vi "Patrick-UTiLIA-Lock.vi"(2 "Reset Filter?":bool, 3 "Sampling Info":cluster{"Fs":dbl[unit], "#S":i32}={"Fs"=55872.0, "#S"=8192}, 4 "Cutoff Freq":dbl[unit]=0.9 format="%.2f", 5 "Filter Type":T1(ring)=enum."Chebyshev", 6 "Unit Reference":dbl[](array[numeric]) format="%.2f", 7 "Noisy Signal":dbl[](array[numeric]) format="%.2f") -> (0 "Multiplied Signal":dbl[](array[numeric]) format="%.2f", 1 "Locked Signal":dbl[](array[numeric]) format="%.2f")   [LabVIEW 2013]
uses:
  <vilib>/Analysis/3filter.llb/Butterworth Filter (DBL).vi
  <vilib>/Analysis/3filter.llb/Chebyshev Filter (DBL).vi
  <vilib>/Analysis/3filter.llb/Inverse Chebyshev Filter (DBL).vi
  <vilib>/Analysis/NI_AALBase.lvlib
panel:
  in  "Attenuation(dB)":dbl=120.0 format="%.2f"
  in  "Filter Order":i32=10
  in  "Passband Ripple(dB)":dbl=0.1 format="%.2f"
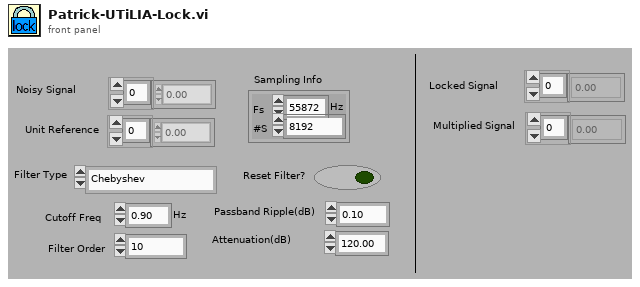
[diagram p1: front panel]
types:
  T1 = enum16{"None", "Butterworth", "Chebyshev", "Inv Chebyshev"}
  T2 = enum32{"Lowpass", "Highpass", "Bandpass", "Bandstop"}
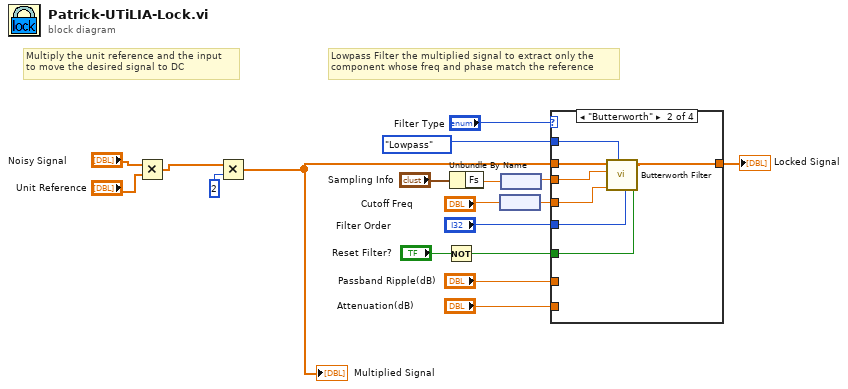
[diagram p0: block diagram]
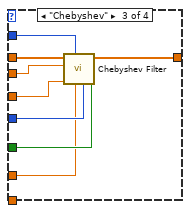
[diagram p3: hidden frame]
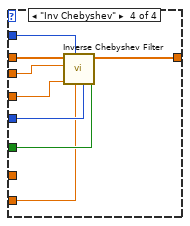
[diagram p4: hidden frame]
diagram:
  # "Lowpass Filter the multiplied signal to extract only the\ncomponent whose freq and phase match the reference"
  # "Multiply the unit reference and the input\nto move the desired signal to DC"
  n1 = Multiply(x="Noisy Signal", y="Unit Reference") -> (x*y=w7:dbl[])
  n2 = Multiply(x=w7, y=2) -> (x*y=w6:dbl[])
  "Multiplied Signal" <- w6
  n3 = Not(x="Reset Filter?") -> (.not. x?=w10:bool)
  n4 = Unbundle By Name("Sampling Info") -> ("Fs"=w1:dbl[unit])
  n5 = node("Cutoff Freq") -> (w3:dbl)
  n6 = node(w1) -> (w4:dbl)
  n7 = case shown="\"Butterworth\"" "Filter Type" {
    tunnel: [w19 w21 w28 w35] -> w11
    tunnel: T2."Lowpass" ("filter type") -> [_ w26 w34 w42]
    tunnel: w3 -> [_ w25 w32 w40]
    tunnel: "Filter Order" -> [_ w24 w31 w39]
    tunnel: w10 -> [_ w23 w30 w38]
    tunnel: w6 -> [w19 w20 w27 w36]
    tunnel: w4 -> [_ w22 w33 w41]
    tunnel: "Attenuation(dB)" -> [_ _ _ w37]
    tunnel: "Passband Ripple(dB)" -> [_ _ w29 _]
    frame "None" {
    }
    frame "Butterworth" {
      n8 = call-poly <vilib>:"Butterworth Filter.vi"("init/cont (init:F)"=w23, "order"=w24, "filter type"=w26, "low cutoff freq: fl"=w25, "sampling freq: fs"=w22, "X"=w20) -> ("Filtered X"=w21:dbl[])  [unwired: 2 in, 1 out]
    }
    frame "Chebyshev" {
      n9 = call-poly <vilib>:"Chebyshev Filter.vi"("init/cont (init:F)"=w30, "order"=w31, "ripple(dB)"=w29, "filter type"=w34, "low cutoff freq: fl"=w32, "sampling freq: fs"=w33, "X"=w27) -> ("Filtered X"=w28:dbl[])  [unwired: 3 in, 1 out]
    }
    frame "Inv Chebyshev" {
      n10 = call-poly <vilib>:"Inverse Chebyshev Filter.vi"("init/cont (init:F)"=w38, "order"=w39, "attenuation (dB)"=w37, "filter type"=w42, "low cutoff freq: fl"=w40, "sampling freq: fs"=w41, "X"=w36) -> ("Filtered X"=w35:dbl[])  [unwired: 3 in, 1 out]
    }
  }
  "Locked Signal" <- w11
